vi "PythonFacade.vi"(0 "Data In":T4, 2 "Display State In":T2, 3 "Container State":T3) -> (6 "Data Out":T4, 7 "Display State Out":T2, 8 "Action":T1)   [LabVIEW 2016, in "uPythonX.xctl"]
uses:
  uPythonX.xctl
  <vilib>/_xctls/Action.ctl
  <vilib>/_xctls/XControlSupport.lvlib
  <vilib>/_xctls/Container State.ctl
  PythonData.ctl
  PythonState.ctl
panel:
  in  "REPL":bool
  out "Port":string
  in  "Help":bool
  in  "Python":T5
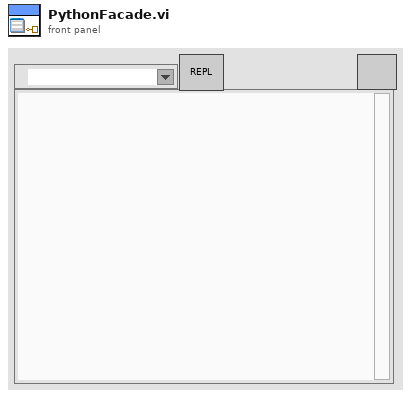
[diagram p1: front panel]
types:
  T1 = typedef "XControlSupport.lvlib/Action.ctl" = cluster{"Data Changed?":bool, "State Changed?":bool, "Action Name":string}
  T2 = typedef "uPythonX.xctl/PythonState.ctl" = cluster{"Numeric":dbl}
  T3 = typedef "XControlSupport.lvlib/Container State.ctl" = cluster{"Indicator?":bool, "Run Mode?":bool, " Refnum":refnum<vi>}
  T4 = typedef "uPythonX.xctl/PythonData.ctl" = cluster{"VISA Refnum in":refnum<visa-resource-name>, "Python Code":string}
  T5 = cluster{"VISA in":refnum<visa-resource-name>, "Code":string}
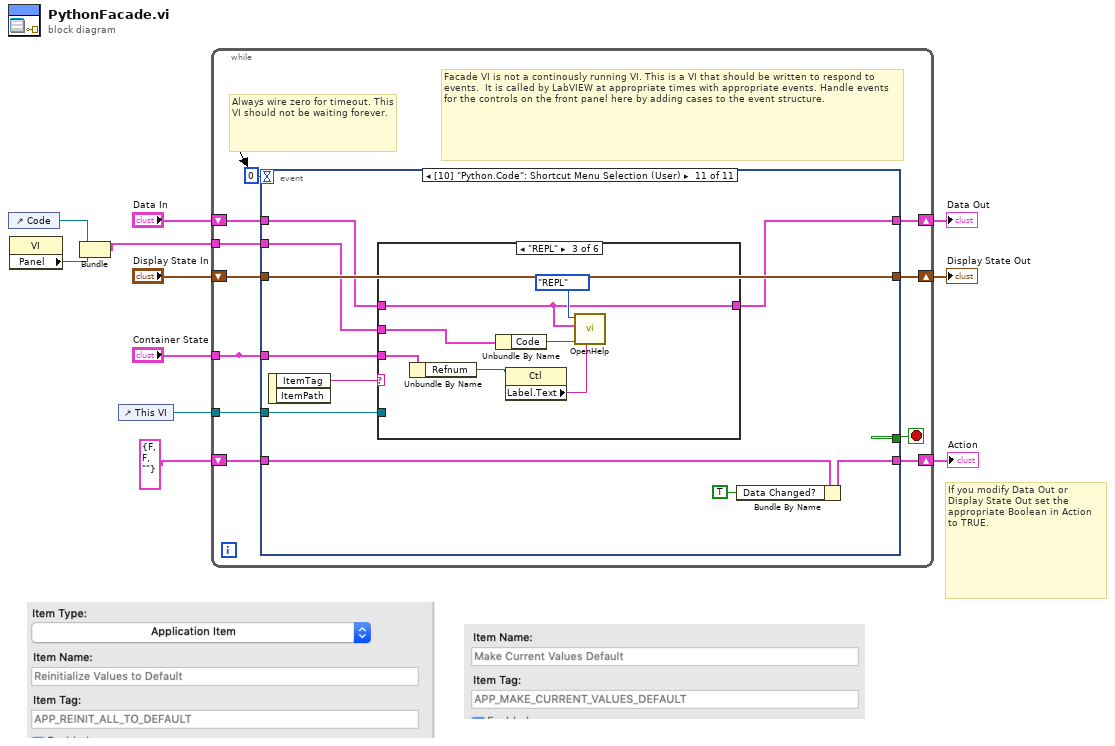
[diagram p0: block diagram]
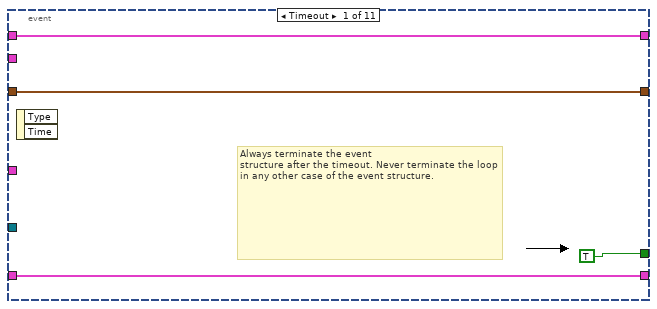
[diagram p2: hidden frame]
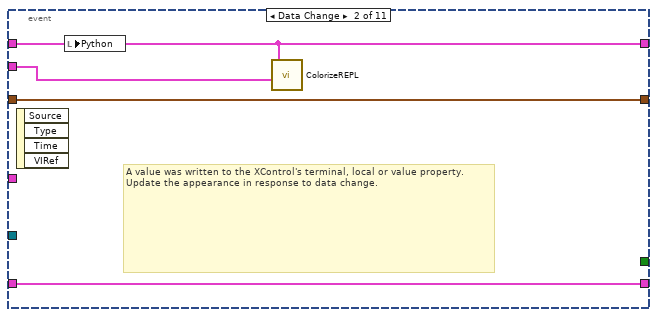
[diagram p3: hidden frame]
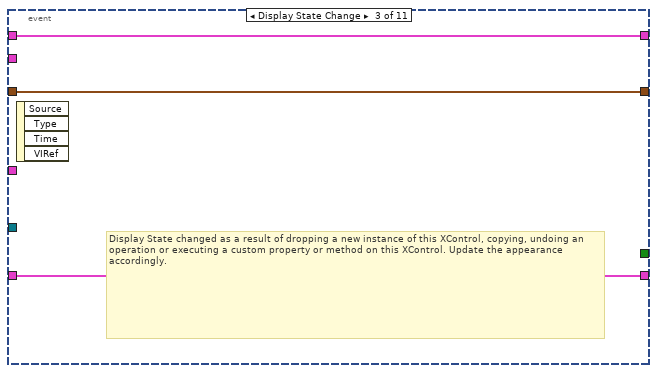
[diagram p4: hidden frame]
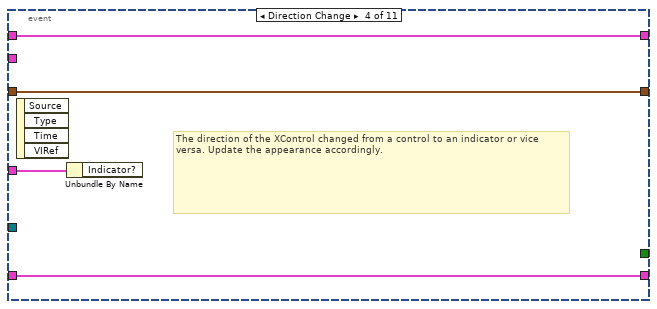
[diagram p5: hidden frame]
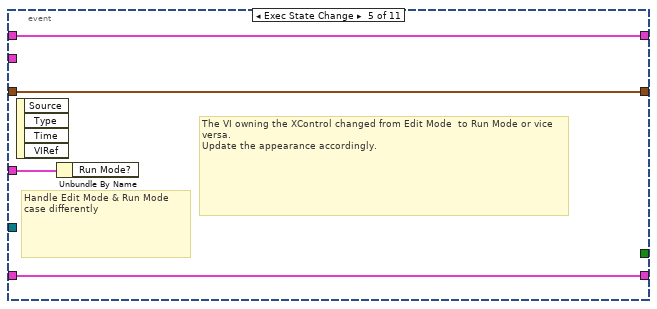
[diagram p6: hidden frame]
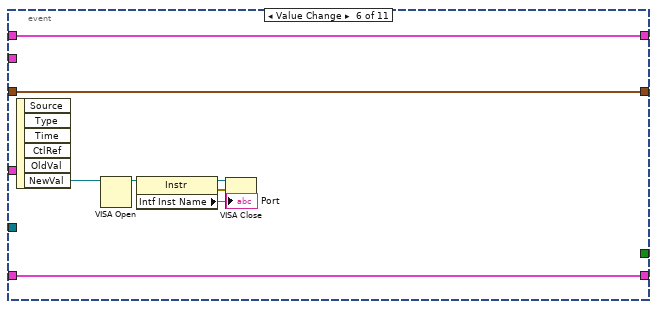
[diagram p7: hidden frame]
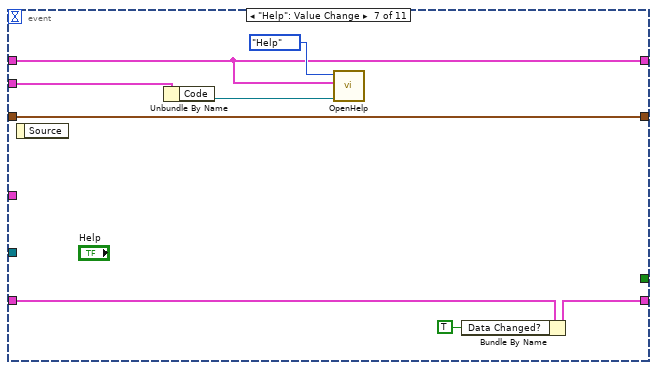
[diagram p8: hidden frame]
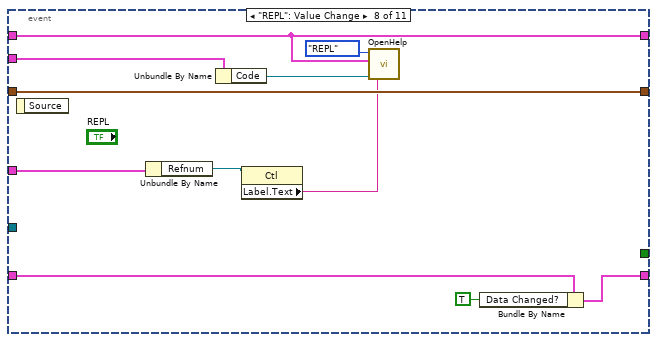
[diagram p9: hidden frame]
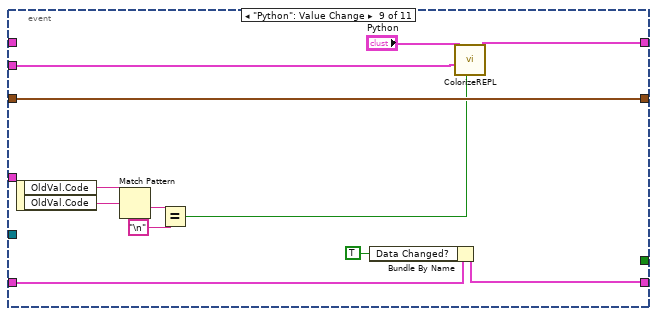
[diagram p10: hidden frame]
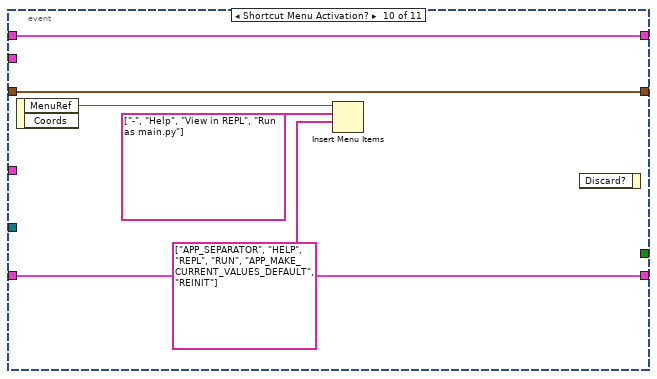
[diagram p11: hidden frame]
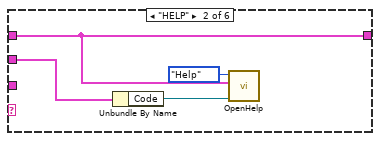
[diagram p13: hidden frame]
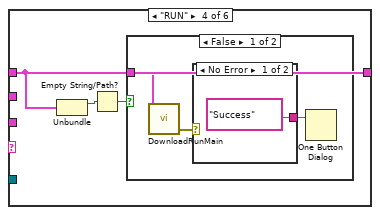
[diagram p14: hidden frame]
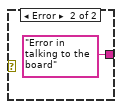
[diagram p15: hidden frame]
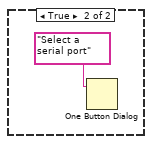
[diagram p16: hidden frame]
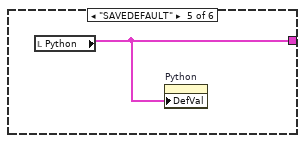
[diagram p17: hidden frame]
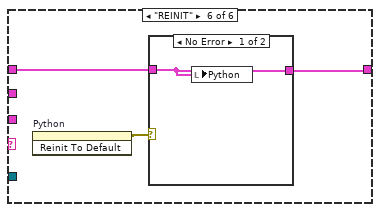
[diagram p18: hidden frame]
diagram:
  # "If you modify Data Out or\nDisplay State Out set the\nappropriate Boolean in Action\nto TRUE."
  n1 = control-ref of="Code"() -> (w3:refnum<vi>)
  n2 = property class="VI"() -> ("Panel"=w2:refnum<vi>)  [unwired: 2 in, 2 out]
  n3 = Bundle("Code"=w3, "Panel"=w2) -> (w1:cluster{"Code":refnum<vi>, "Panel":refnum<vi>})  [unwired: 1 in]
  n4 = control-ref of="This VI"() -> (w4:refnum<vi>)
  n5 = while {
    shift-right: [w21] -> w8
    shift-left: "Display State In" -> [w22]
    tunnel: "Container State" -> [w12]
    shift-right: [w17] -> w11
    shift-left: "Data In" -> [w18]
    shift-right: [w15] -> w6
    shift-left: T1 {"Data Changed?"=FALSE, "State Changed?"=FALSE, "Action Name"=""} ("Action") -> [w16]
    tunnel: w4 -> [w14]
    tunnel: w1 -> [w13]
    tunnel: [w12] -> _
    stop <- w20 stop-if-true
    # "Facade VI is not a continously running VI. This is a VI that should be written to respond to events.  It is called by LabVIEW at appropriate times with appropriate events. Handle events for the controls on the front panel here by adding cases to the event structure."
    # "Always wire zero for timeout. This\nVI should not be waiting forever."
    n6 = event shown="[10] \"Python.Code\": Shortcut Menu Selection (User)" {
      selector: _ -> [_ _ _ _ _ _ _ _ _ _ _]
      dyn-events: _ -> [_ _ _ _ _ _ _ _ _ _ _]
      timeout: 0 -> [_ _ _ _ _ _ _ _ _ _ _]
      tunnel: w22 -> [w24 w30 w33 w36 w40 w49 w57 w68 w80 w86 w96]
      tunnel: [w24 w30 w33 w36 w40 w49 w57 w68 w80 w86 w96] -> w21
      tunnel: [TRUE _ _ _ _ _ _ _ _ _ _] -> w20
      tunnel: w12 -> [_ _ _ w37 w41 _ _ w59 _ _ w87]
      tunnel: w18 -> [w23 w27 w31 w35 w39 w48 w52 w62 _ w85 w95]
      tunnel: [w23 w27 w31 w35 w39 w48 w52 w62 w75 w85 w94] -> w17
      tunnel: [w25 w29 w32 w34 w38 w47 w54 w65 w77 w84 w89] -> w15
      tunnel: w16 -> [w25 w29 w32 w34 w38 w47 w55 w66 w79 w84 w90]
      tunnel: w14 -> [_ _ _ _ _ _ _ _ _ _ w92]
      tunnel: w13 -> [_ w28 _ _ _ _ w51 w64 w74 _ w88]
      event Timeout {
        # "Always terminate the event\nstructure after the timeout. Never terminate the loop in any other case of the event structure."
        n7 = event-data() -> ()  [unwired: 1 in, 2 out]
      }
      event Data Change {
        # "A value was written to the XControl's terminal, local or value property.\nUpdate the appearance in response to data change."
        n8 = event-data() -> ()  [unwired: 1 in, 4 out]
        n9 = local write "Python"(w27) -> ()
        n10 = call "ColorizeREPL.vi"("Data In"=w27, "refs"=w28) -> ()  [unwired: 8 in, 1 out]
      }
      event Display State Change {
        # "Display State changed as a result of dropping a new instance of this XControl, copying, undoing an operation or executing a custom property or method on this XControl. Update the appearance accordingly."
        n11 = event-data() -> ()  [unwired: 1 in, 4 out]
      }
      event Direction Change {
        # "The direction of the XControl changed from a control to an indicator or vice versa. Update the appearance accordingly."
        n12 = event-data() -> ()  [unwired: 1 in, 4 out]
        n13 = Unbundle By Name(w37) -> ()  [unwired: 1 out]
      }
      event Exec State Change {
        # "The VI owning the XControl changed from Edit Mode  to Run Mode or vice versa.\nUpdate the appearance accordingly."
        # "Handle Edit Mode & Run Mode\ncase differently"
        n14 = event-data() -> ()  [unwired: 1 in, 4 out]
        n15 = Unbundle By Name(w41) -> ()  [unwired: 1 out]
      }
      event "Python.VISA in": Value Change {
        n16 = event-data() -> ("NewVal"=w43:refnum<visa-resource-name>)  [unwired: 1 in, 5 out]
        n17 = VISA Open(VISA resource name=w43) -> (VISA resource name=w44:refnum<visa-resource-name>)  [unwired: 4 in, 1 out]
        n18 = property class="Instr"(reference=w44) -> (reference out=w46:refnum<visa-resource-name>, error out=w45:errorcluster, "Intf Inst Name"=→"Port":string)  [unwired: 1 in]
        n19 = VISA Close(VISA resource name=w46, error in (no error)=w45) -> ()  [unwired: 1 out]
      }
      event "Help": Value Change {
        n20 = event-data() -> ()  [unwired: 1 in, 1 out]
        n21 = Unbundle By Name(w51) -> ("Code"=w50:refnum<vi>)
        n22 = call "OpenHelp.vi"("Code Ref"=w50, "Microprocessor in"=w52, "Dialog"=enum16{"REPL", "Help"}."Help") -> ()  [unwired: 9 in]
        n23 = Bundle By Name(cluster=w55, "Data Changed?"=TRUE) -> (w54:T1)
      }
      event "REPL": Value Change {
        n24 = event-data() -> ()  [unwired: 1 in, 1 out]
        n25 = Unbundle By Name(w59) -> ("Refnum"=w60:refnum<vi>)
        n26 = Unbundle By Name(w64) -> ("Code"=w61:refnum<vi>)
        n27 = property class="Ctl"(reference=w60) -> ("Label.Text"=w58:string)  [unwired: 1 in, 2 out]
        n28 = call "OpenHelp.vi"("Control Name"=w58, "Code Ref"=w61, "Microprocessor in"=w62, "Dialog"=enum16{"REPL", "Help"}."REPL") -> ()  [unwired: 8 in]
        n29 = Bundle By Name(cluster=w66, "Data Changed?"=TRUE) -> (w65:T1)
      }
      event "Python": Value Change {
        n30 = event-data() -> ("OldVal.Code"=w73:string, "OldVal.Code"=w72:string)  [unwired: 1 in]
        n31 = Match Pattern(string=w73, regular expression=w72) -> (after substring=w70:string)  [unwired: 1 in, 3 out]
        n32 = Equal?(x=w70, y="\n") -> (x = y?=w71:bool)
        n33 = Bundle By Name(cluster=w79, "Data Changed?"=TRUE) -> (w77:T1)
        n34 = call "ColorizeREPL.vi"("Data In"="Python", "refs"=w74, "Add Spaces?"=w71) -> ("Data out"=w75:T4)  [unwired: 7 in]
      }
      event "Python.Code": Shortcut Menu Activation? {
        n35 = event-data() -> ("MenuRef"=w81:refnum<k9>)  [unwired: 1 in, 1 out]
        n36 = Insert Menu Items(7:string[] ["APP_SEPARATOR", "HELP", "REPL", "RUN", "APP_MAKE_CURRENT_VALUES_DEFAULT", "REINIT"], 8:string[] ["-", "Help", "View in REPL", "Run as main.py"], 9:w81) -> ()  [unwired: 3 in, 3 out]
        n37 = event-data() -> ()  [unwired: 2 in, 1 out]
      }
      event "Python.Code": Shortcut Menu Selection (User) {
        n38 = event-data() -> ("ItemTag"=w93:string)  [unwired: 1 in, 1 out]
        n39 = case shown="\"REPL\"" w93 {
          tunnel: w95 -> [w97 w101 w107 w111 _ w120]
          tunnel: [w97 w101 w107 w111 w118 w119] -> w94
          tunnel: w92 -> [_ _ _ _ _ _]
          tunnel: w88 -> [_ w99 w106 _ _ _]
          tunnel: w87 -> [_ _ w103 _ _ _]
          frame Default {
          }
          frame "HELP" {
            n40 = Unbundle By Name(w99) -> ("Code"=w98:refnum<vi>)
            n41 = call "OpenHelp.vi"("Code Ref"=w98, "Microprocessor in"=w101, "Dialog"=enum16{"REPL", "Help"}."Help") -> ()  [unwired: 9 in]
          }
          frame "REPL" {
            n42 = Unbundle By Name(w103) -> ("Refnum"=w104:refnum<vi>)
            n43 = Unbundle By Name(w106) -> ("Code"=w105:refnum<vi>)
            n44 = property class="Ctl"(reference=w104) -> ("Label.Text"=w102:string)  [unwired: 1 in, 2 out]
            n45 = call "OpenHelp.vi"("Control Name"=w102, "Code Ref"=w105, "Microprocessor in"=w107, "Dialog"=enum16{"REPL", "Help"}."REPL") -> ()  [unwired: 8 in]
          }
          frame "RUN" {
            n46 = Unbundle(w111) -> ("VISA Refnum in"=w110:refnum<visa-resource-name>)  [unwired: 1 out]
            n47 = Empty String/Path?(string/path=w110) -> (empty?=w109:bool)
            n48 = case shown="False" w109 {
              tunnel: w111 -> [w114 _]
              frame False {
                n49 = call "DownloadRunMain.vi"("uPythonX"=w114) -> ("error out"=w112:errorcluster)  [unwired: 8 in, 2 out]
                n50 = case shown="No Error" w112 {
                  tunnel: ["Success" ("message") "Error in talking to the board" ("message")] -> w113
                  frame No Error {
                  }
                  frame Error {
                  }
                }
                n51 = One Button Dialog(message=w113) -> ()  [unwired: 1 in, 1 out]
              }
              frame True {
                n52 = One Button Dialog(message="Select a serial port") -> ()  [unwired: 1 in, 1 out]
              }
            }
          }
          frame "SAVEDEFAULT" {
            n53 = local read "Python"() -> (w118:T5)
            n54 = property on="Python" class="Clust (strict)"("DefVal"=w118) -> ()  [unwired: 2 in, 2 out]
          }
          frame "REINIT" {
            n55 = invoke on="Python" class="Clust (strict)" method="Reinit To Default"() -> (error out=w121:errorcluster)  [unwired: 3 in, 2 out]
            n56 = case shown="No Error" w121 {
              tunnel: w120 -> [w122 w123]
              tunnel: [w122 w123] -> w119
              frame No Error {
                n57 = local write "Python"(w122) -> ()
              }
              frame Error {
              }
            }
          }
        }
        n58 = Bundle By Name(cluster=w90, "Data Changed?"=TRUE) -> (w89:T1)
      }
    }
  }
  "Display State Out" <- w8
  "Data Out" <- w11
  "Action" <- w6
